vi "18-Add.vi"(10 "Snailfish Number y":string, 11 "Snailfish Number x":string) -> (3 "Snailfish Number x+y":string)   [LabVIEW 2019, in "18.lvlib"]
uses:
  18.lvlib
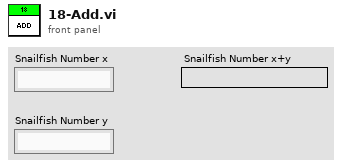
[diagram p1: front panel]
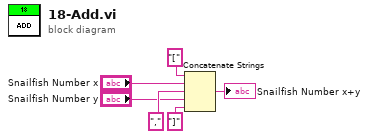
[diagram p0: block diagram]
diagram:
  n1 = Concatenate Strings("[", "Snailfish Number x", ",", "Snailfish Number y", "]") -> (→"Snailfish Number x+y":string)
